vi "Commande ST5V2.vi"(4 "error in (no error)":errorcluster, 6 "Commande":string, 7 "Port COM":refnum<visa-resource-name>) -> (0 "error out":errorcluster, 1 "Read":u32, 2 "Réponse":string, 3 "Port Out":refnum<visa-resource-name>)   [LabVIEW 2019]
doc: "Ce Vi envoie les chaînes de commande au contrôlleur de moteur ST5-Q et vérifie si une réponse se trouve dans le buffer du port série"
uses:
  <vilib>/Instr/_visa.llb/VISA Configure Serial Port (Instr).vi
panel:
  out "Sent":u32
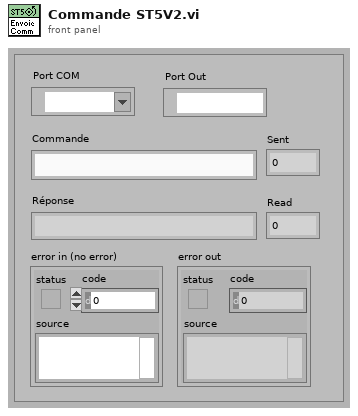
[diagram p1: front panel]
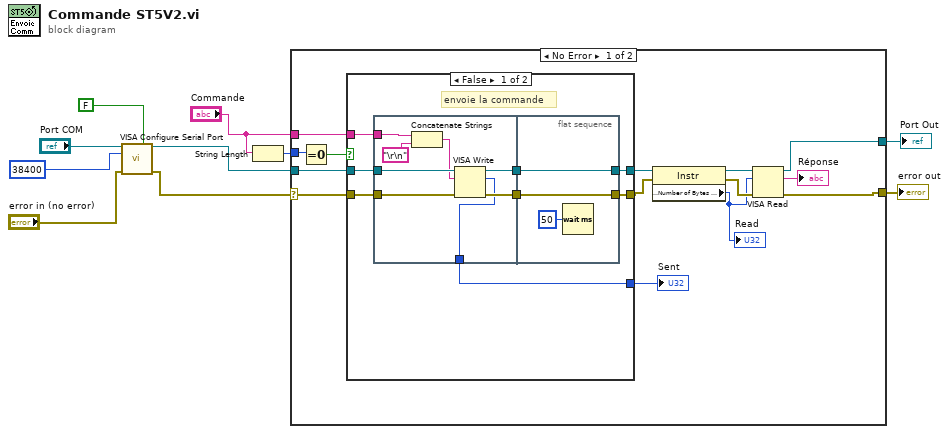
[diagram p0: block diagram]
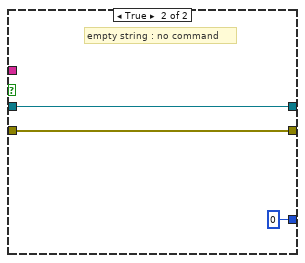
[diagram p2: hidden frame]
diagram:
  n1 = call-poly "VISA Configure Serial Port"("VISA resource name"="Port COM", "Enable Termination\nChar (T)"=FALSE ("Enable Termination\nChar (T)"), "baud rate (9600)"=u32 38400, "error in (no error)"="error in (no error)") -> ("VISA resource name out"=w5:refnum<visa-resource-name>, "error out"=w1:errorcluster)  [unwired: 10 in]
  n2 = String Length(string="Commande") -> (length=w8:i32)
  n3 = case shown="No Error" w1 {
    selector: w1 -> [w23 w48]
    tunnel: w5 -> [w24 w47]
    tunnel: [w22 w48] -> w10
    tunnel: "Commande" -> [w21 _]
    tunnel: w8 -> [w18 _]
    tunnel: [w16 w47] -> w7
    frame No Error {
      n4 = Equal To 0?(x=w18) -> (x = 0?=w17:bool)
      n5 = case shown="False" w17 {
        tunnel: w23 -> [w32 w45]
        tunnel: w24 -> [w31 w46]
        tunnel: [w30 w45] -> w20
        tunnel: [w29 w46] -> w19
        tunnel: w21 -> [w26 _]
        tunnel: [w25 u32 0 ("return count")] -> w11
        frame False {
          # "envoie la commande"
          n6 = flat-sequence {
            tunnel: w32 -> [w40]
            tunnel: w31 -> [w38]
            tunnel: w26 -> [w35]
            tunnel: [w37] -> w28
            tunnel: [w36] -> w27
            tunnel: [w33] -> w25
            tunnel: [w42] -> w29
            tunnel: [w43] -> w30
            tunnel: w28 -> [w43]
            tunnel: w27 -> [w42]
            frame #0 {
              n7 = Concatenate Strings(w35, "\r\n") -> (w34:string)
              n8 = VISA Write(VISA resource name=w38, write buffer=w34, error in (no error)=w40) -> (VISA resource name out=w36:refnum<visa-resource-name>, return count=w33:u32, error out=w37:errorcluster)
            }
            frame #1 {
              n9 = Wait (ms)(milliseconds to wait=u32 50) -> ()  [unwired: 1 out]
            }
          }
        }
        frame True {
          # "empty string : no command"
        }
      }
      "Sent" <- w11
      n10 = property class="Instr"(reference=w19, error in=w20) -> (reference out=w13:refnum<visa-resource-name>, error out=w14:errorcluster, "Serial Settings:Number of Bytes at Serial Port"=w12:u32)
      "Read" <- w12
      n11 = VISA Read(VISA resource name=w13, byte count=w12, error in (no error)=w14) -> (VISA resource name out=w16:refnum<visa-resource-name>, read buffer=→"Réponse":string, error out=w22:errorcluster)  [unwired: 1 out]
    }
    frame Error {
    }
  }
  "error out" <- w10
  "Port Out" <- w7
